vi "Sys config-Maintain hidden config values.vi"(10 "New System Configuration":T1={"Ethernet opened"=FALSE, "Ethernet Port"=3, "Ctrl FPGA available"=FALSE, "Ctrl FPGA Clock (MHz)"=240.0, "Ctrl system MAC address"="", "Control system.Network adapter name"="", "AOD 1 Amplitude"=0, "AOD 2 Amplitude"=0, "AOD 3 Amplitude"=0, "AOD 4 Amplitude"=0, "Data Time Interval (ns)"=0.0, "T0 (ns)"=0.0, "Ta (ns)"=0.0} {"Ctrl FPGA Clock (MHz)" min=80.0 max=500.0 step=1.0; "Data Time Interval (ns)" min=0.0 max=2048.0 step=1.0; "Ta (ns)" min=0.0 max=2048.0 step=1.0; "T0 (ns)" min=0.0 max=2048.0 step=1.0; "AOD 4 Amplitude" min=0 max=2048 step=1; "AOD 3 Amplitude" min=0 max=2048 step=1; "AOD 2 Amplitude" min=0 max=2048 step=1; "AOD 1 Amplitude" min=0 max=2048 step=1}, 11 "Existing System Configuration":T2={"XY Stage"={"COM port"="", "XY stage available"=FALSE}, "DAQ FPGA"={"Ref"=refnum, "Target"="RIO0", "Clock Freq (MHz) "=200.0, "input card type"=enum."AC Card", "Samples Wait after Trigger"=5080, "AOD fill"=4900, "StartupDelay"=0, "Slip Cycle (clock cycles)"=600000, "Add Cycle"=TRUE}, "Control system"={"Ethernet opened"=FALSE, "Ethernet Port"=3, "Ctrl FPGA available"=FALSE, "Ctrl FPGA Clock (MHz)"=240.0, "Ctrl system MAC address"="", "Control system.Network adapter name"="", "AOD 1 Amplitude"=0, "AOD 2 Amplitude"=0, "AOD 3 Amplitude"=0, "AOD 4 Amplitude"=0, "Data Time Interval (ns)"=0.0, "T0 (ns)"=0.0, "Ta (ns)"=0.0}, "Encoder"={"IP address"="224.0.1.103", "Port"=7000, "Encoder available"=FALSE, "Wheel radius (cm)"=16.0}, "DAQmx Chan"={"Pockels AO"="", "Hard shutter AO"="", "PMT AOs"="", "Power meter AI"=""}, "Computer MAC address"="", "Cam VidRec"={"DO flag-Video record"="", "DO flag-Trial start"="", "VidRec available"=FALSE}, "Externalise Triggers"=FALSE, "Laser wavelength (nm)"=920.0} {"Laser wavelength (nm)" min=800.0 max=1080.0 step=1.0; "Encoder"."Wheel radius (cm)" format="%#_13g"; "Control system"."Ctrl FPGA Clock (MHz)" min=80.0 max=500.0 step=1.0; "Control system"."Data Time Interval (ns)" min=0.0 max=2048.0 step=1.0; "Control system"."Ta (ns)" min=0.0 max=2048.0 step=1.0; "Control system"."T0 (ns)" min=0.0 max=2048.0 step=1.0; "Control system"."AOD 4 Amplitude" min=0 max=2048 step=1; "Control system"."AOD 3 Amplitude" min=0 max=2048 step=1; "Control system"."AOD 2 Amplitude" min=0 max=2048 step=1; "Control system"."AOD 1 Amplitude" min=0 max=2048 step=1}) -> (3 "Updated System Configuration":T1={"Ethernet opened"=FALSE, "Ethernet Port"=3, "Ctrl FPGA available"=FALSE, "Ctrl FPGA Clock (MHz)"=240.0, "Ctrl system MAC address"="", "Control system.Network adapter name"="", "AOD 1 Amplitude"=0, "AOD 2 Amplitude"=0, "AOD 3 Amplitude"=0, "AOD 4 Amplitude"=0, "Data Time Interval (ns)"=0.0, "T0 (ns)"=0.0, "Ta (ns)"=0.0} {"Ctrl FPGA Clock (MHz)" min=80.0 max=500.0 step=1.0; "Data Time Interval (ns)" min=0.0 max=2048.0 step=1.0; "Ta (ns)" min=0.0 max=2048.0 step=1.0; "T0 (ns)" min=0.0 max=2048.0 step=1.0; "AOD 4 Amplitude" min=0 max=2048 step=1; "AOD 3 Amplitude" min=0 max=2048 step=1; "AOD 2 Amplitude" min=0 max=2048 step=1; "AOD 1 Amplitude" min=0 max=2048 step=1})   [LabVIEW 2013]
uses:
  Typedefs/Sys Configuration.ctl
  Typedefs/XY Stage config cluster.ctl
  Typedefs/DAQ FPGA config cluster.ctl
  RIG-SPECIFIC FILES/FPGA Refs/FPGA Ref.ctl
  <vilib>/userdefined/High Color/nirio_resource_hc.ctl
  Typedefs/FPGA input type AC-DC.ctl
  Typedefs/CTRL system config cluster.ctl
  Typedefs/Encoder config cluster.ctl
  Typedefs/DAQmx physical channels cluster.ctl
  Typedefs/Cam VidRec HW config setup cluster.ctl
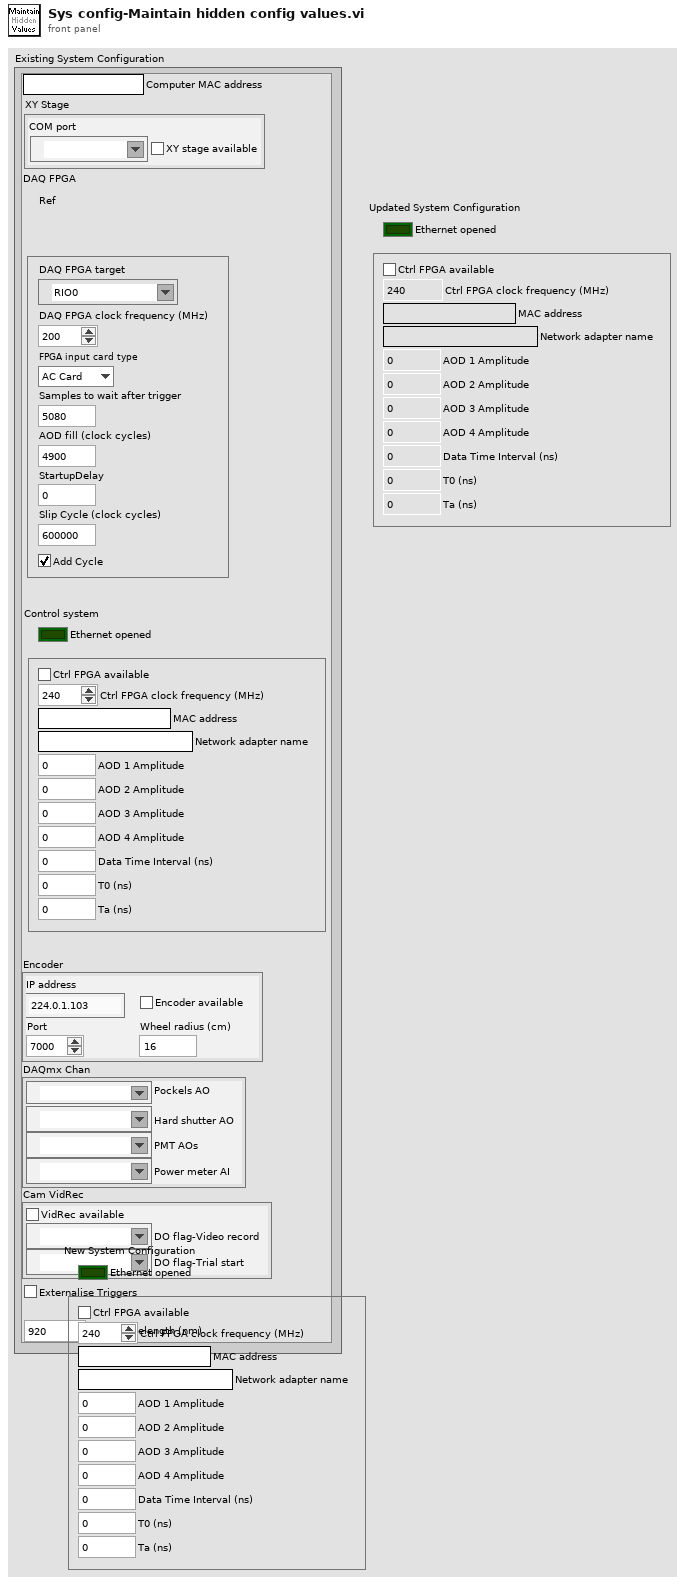
[diagram p1: front panel]
types:
  T1 = typedef "CTRL system config cluster.ctl" = cluster{"Ethernet opened":bool, "Ethernet Port":u32, "Ctrl FPGA available":bool, "Ctrl FPGA Clock (MHz)":dbl, "Ctrl system MAC address":string, "Control system.Network adapter name":string, "AOD 1 Amplitude":i16, "AOD 2 Amplitude":i16, "AOD 3 Amplitude":i16, "AOD 4 Amplitude":i16, "Data Time Interval (ns)":dbl, "T0 (ns)":dbl, "Ta (ns)":dbl}
  T2 = typedef "Sys Configuration.ctl" = cluster{"XY Stage":T3, "DAQ FPGA":T4, "Control system":T1, "Encoder":T8, "DAQmx Chan":T9, "Computer MAC address":string, "Cam VidRec":T10, "Externalise Triggers":bool, "Laser wavelength (nm)":dbl}
  T3 = typedef "XY Stage config cluster.ctl" = cluster{"COM port":refnum<visa-resource-name>, "XY stage available":bool}
  T4 = typedef "DAQ FPGA config cluster.ctl" = cluster{"Ref":T5, "Target":T6, "Clock Freq (MHz) ":dbl, "input card type":T7, "Samples Wait after Trigger":u16, "AOD fill":u16, "StartupDelay":i32, "Slip Cycle (clock cycles)":u32, "Add Cycle":bool}
  T5 = typedef "FPGA Ref.ctl" = refnum<k20>
  T6 = typedef "nirio_resource_hc.ctl" = tag
  T7 = typedef "FPGA input type AC-DC.ctl" = enum16{"AC Card", "DC Card"}
  T8 = typedef "Encoder config cluster.ctl" = cluster{"IP address":string, "Port":u16, "Encoder available":bool, "Wheel radius (cm)":dbl}
  T9 = typedef "DAQmx physical channels cluster.ctl" = cluster{"Pockels AO":tag, "Hard shutter AO":tag, "PMT AOs":tag, "Power meter AI":tag}
  T10 = typedef "Cam VidRec HW config setup cluster.ctl" = cluster{"DO flag-Video record":tag, "DO flag-Trial start":tag, "VidRec available":bool}
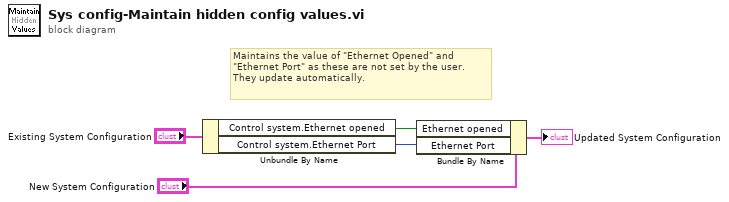
[diagram p0: block diagram]
diagram:
  # "Maintains the value of \"Ethernet Opened\" and \"Ethernet Port\" as these are not set by the user.\nThey update automatically."
  n1 = Unbundle By Name("Existing System Configuration") -> ("Control system.Ethernet opened"=w5:bool, "Control system.Ethernet Port"=w1:u32)
  n2 = Bundle By Name(cluster="New System Configuration", "Ethernet opened"=w5, "Ethernet Port"=w1) -> (→"Updated System Configuration":T1)
